vi "Move.vi"(5 "Force":bool, 7 "Valve":string, 10 "max time":i32=26, 11 "Volcano in":refnum<class "Volcano.lvclass">=refnum) -> (1 "Finished?":bool=TRUE, 2 "# elements in queue":i32, 3 "Volcano out":refnum<class "Volcano.lvclass">)   [LabVIEW 2023, in "d16.lvlib" / "Volcano.lvclass"]
uses:
  Volcano.lvclass
  Volcano.lvclass/Volcano.ctl
  <vilib>/Utility/miscctls.llb/LVMapReplaceAction.ctl
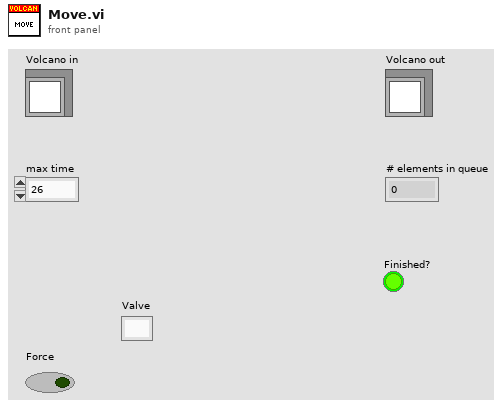
[diagram p1: front panel]
types:
  T1 = typedef "LVMapReplaceAction.ctl" = enum32{"Modify Entry only if found", "Add or Modify Entry", "Delete Entry"}
  T2 = cluster{"Current Valve":string, "Unopened Valves":string[], "Cumulative Pressure Released":u64, "Time":i32}
  T3 = map{string, cluster{"Flow Rate":i32, "Routes":string[], "Route Time":i32[]}}
  T4 = cluster{"Flow Rate":i32, "Routes":string[], "Route Time":i32[]}
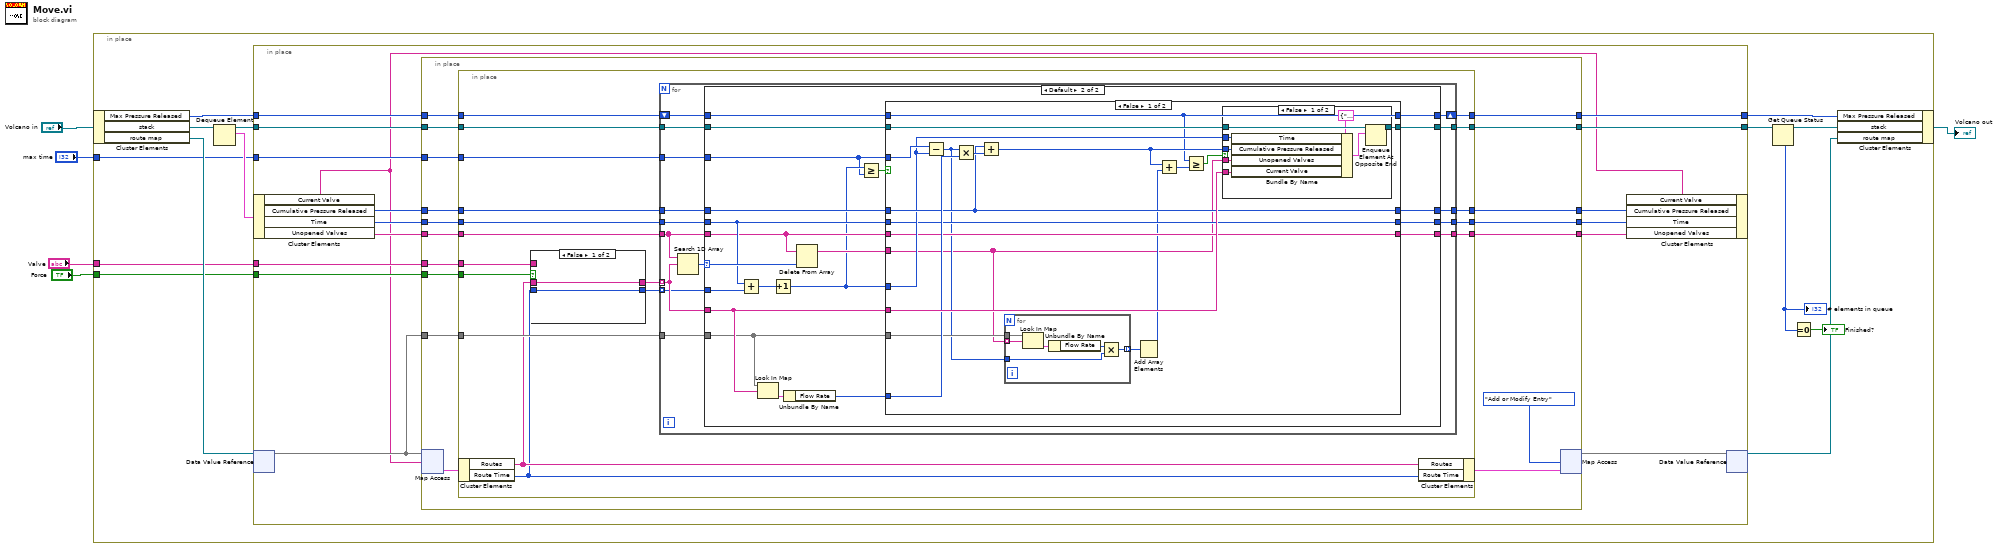
[diagram p0: block diagram]
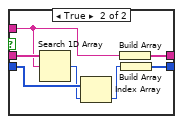
[diagram p2: hidden frame]
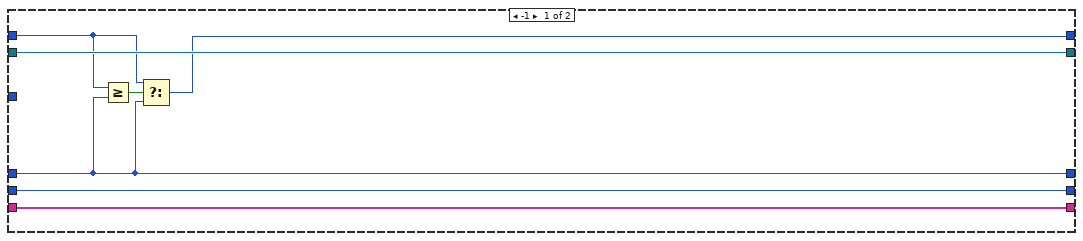
[diagram p3: hidden frame]
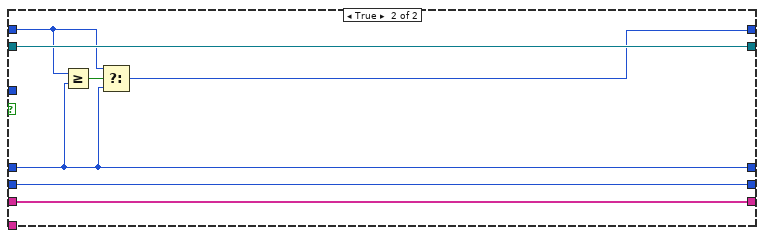
[diagram p5: hidden frame]
diagram:
  n1 = in-place {
    in-place-border: "max time" -> [w15]
    in-place-border: "Force" -> [w7]
    in-place-border: "Valve" -> [w6]
    n2 = in-place-cluster #1("Volcano in") -> ("Max Pressure Released"=w13:u64, "stack"=w19:refnum<queue>, "route map"=w17:refnum<data-value>)
    n3 = Dequeue Element(queue=w19) -> (queue out=w18:refnum<queue>, element=w16:T2)  [unwired: 2 in, 2 out]
    n4 = in-place {
      in-place-border: w18 -> [w35]
      in-place-border: w15 -> [w34]
      in-place-border: [w33] -> w11
      in-place-border: w13 -> [w31]
      in-place-border: [w30] -> w12
      in-place-border: w7 -> [w28]
      in-place-border: w6 -> [w27]
      n5 = in-place-cluster #2(w16) -> ("Current Valve"=w20:string, "Cumulative Pressure Released"=w24:u64, "Time"=w22:i32, "Unopened Valves"=w25:string[])
      n6 = in-place-dvr #3(w17) -> (w29:T3)  [unwired: 1 out]
      n7 = in-place {
        in-place-border: w35 -> [w50]
        in-place-border: w24 -> [w51]
        in-place-border: w34 -> [w44]
        in-place-border: [w49] -> w33
        in-place-border: w22 -> [w45]
        in-place-border: w31 -> [w43]
        in-place-border: [w42] -> w30
        in-place-border: w25 -> [w46]
        in-place-border: w29 -> [w41]
        in-place-border: w28 -> [w40]
        in-place-border: w27 -> [w39]
        in-place-border: [w38] -> w26
        in-place-border: [w37] -> w21
        in-place-border: [w36] -> w23
        n8 = in-place-map #4(w29, w20) -> (w52:T4)  [unwired: 1 in, 1 out]
        n9 = in-place {
          in-place-border: w45 -> [w66]
          in-place-border: w44 -> [w64]
          in-place-border: w51 -> [w65]
          in-place-border: w50 -> [w70]
          in-place-border: [w69] -> w49
          in-place-border: w46 -> [w67]
          in-place-border: w43 -> [w68]
          in-place-border: [w63] -> w42
          in-place-border: w41 -> [w62]
          in-place-border: w40 -> [w61]
          in-place-border: w39 -> [w56]
          in-place-border: [w55] -> w38
          in-place-border: [w54] -> w37
          in-place-border: [w53] -> w36
          n10 = in-place-cluster #5(w52) -> ("Routes"=w60:string[], "Route Time"=w59:i32[])
          n11 = case shown="False" w61 {
            tunnel: w60 -> [w72 w78]
            tunnel: w59 -> [w71 w76]
            tunnel: [w72 w79] -> w58
            tunnel: [w71 w73] -> w57
            tunnel: w56 -> [_ w77]
            frame False {
            }
            frame True {
              n12 = Search 1D Array(1D array=w78, element=w77) -> (index of element=w75:i32)  [unwired: 1 in]
              n13 = Index Array(array=w76, index=w75) -> (element=w74:i32)
              n14 = Build Array(w77) -> (w79:string[])
              n15 = Build Array(w74) -> (w73:i32[])
            }
          }
          n16 = for {
            tunnel: w70 -> [w94]
            tunnel: [w93] -> w69
            tunnel: w67 -> [w92]
            tunnel: w66 -> [w90]
            tunnel: w65 -> [w87]
            tunnel: w64 -> [w88]
            shift-right: [w86] -> w63
            shift-left: w68 -> [w89]
            tunnel: w62 -> [w85]
            tunnel: w58 -> [w84] mode=indexing
            tunnel: w57 -> [w83] mode=indexing
            tunnel: [w82] -> w55
            tunnel: [w81] -> w54
            tunnel: [w80] -> w53
            n17 = Search 1D Array(1D array=w92, element=w84) -> (index of element=w91:i32)  [unwired: 1 in]
            n18 = case shown="Default" w91 {
              selector: w91 -> [_ w120]
              tunnel: w94 -> [w101 w122]
              tunnel: [w101 w121] -> w93
              tunnel: w92 -> [w95 w107]
              tunnel: w90 -> [w96 w109]
              tunnel: w83 -> [_ w118]
              tunnel: w89 -> [w99 w116]
              tunnel: w88 -> [_ w103]
              tunnel: w87 -> [w97 w115]
              tunnel: [w100 w114] -> w86
              tunnel: w85 -> [_ w102]
              tunnel: w84 -> [_ w113]
              tunnel: [w95 w106] -> w82
              tunnel: [w96 w108] -> w81
              tunnel: [w97 w110] -> w80
              frame -1 {
                n19 = Greater Or Equal?(x=w99, y=w97) -> (x >= y?=w98:bool)
                n20 = Select(t=w99, s=w98, f=w97) -> (s? t:f=w100:u64)
              }
              frame Default {
                n21 = Add(x=w109, y=w118) -> (x+y=w105:i32)
                n22 = Look In Map(map=w102, key=w113) -> (value=w112:T4)  [unwired: 1 in, 1 out]
                n23 = Increment(x=w105) -> (x+1=w104:i32)
                n24 = Unbundle By Name(w112) -> ("Flow Rate"=w111:i32)
                n25 = Delete From Array(array=w107, index=w120) -> (array with subset deleted=w119:string[])  [unwired: 1 in, 1 out]
                n26 = Greater Or Equal?(x=w104, y=w103) -> (x >= y?=w117:bool)
                n27 = case shown="False" w117 {
                  tunnel: w122 -> [w141 w163]
                  tunnel: [w140 w163] -> w121
                  tunnel: w119 -> [w123 _]
                  tunnel: w113 -> [w139 _]
                  tunnel: w116 -> [w125 w162]
                  tunnel: w111 -> [w138 _]
                  tunnel: w104 -> [w134 _]
                  tunnel: w103 -> [w137 _]
                  tunnel: w115 -> [w135 w157]
                  tunnel: [w125 w161] -> w114
                  tunnel: [w135 w157] -> w110
                  tunnel: w107 -> [w132 w159]
                  tunnel: w109 -> [w133 w160]
                  tunnel: [w133 w160] -> w108
                  tunnel: [w132 w159] -> w106
                  tunnel: w102 -> [w131 _]
                  frame False {
                    n28 = Subtract(x=w137, y=w134) -> (x-y=w130:i32)
                    n29 = Multiply(x=w130, y=w138) -> (x*y=w136:i32)
                    n30 = Add(x=w135, y=w136) -> (x+y=w127:u64)
                    n31 = for {
                      tunnel: w123 -> [w156] mode=indexing
                      tunnel: w131 -> [w155]
                      tunnel: w130 -> [w152]
                      tunnel: [w151] -> w129 mode=indexing
                      n32 = Look In Map(map=w155, key=w156) -> (value=w154:T4)  [unwired: 1 in, 1 out]
                      n33 = Unbundle By Name(w154) -> ("Flow Rate"=w153:i32)
                      n34 = Multiply(x=w153, y=w152) -> (x*y=w151:i32)
                    }
                    n35 = Add Array Elements(numeric array=w129) -> (sum=w128:i32)
                    n36 = Add(x=w127, y=w128) -> (x+y=w126:u64)
                    n37 = Greater Or Equal?(x=w125, y=w126) -> (x >= y?=w124:bool)
                    n38 = case shown="False" w124 {
                      tunnel: w141 -> [w149 w150]
                      tunnel: [w147 w150] -> w140
                      tunnel: w139 -> [w145 _]
                      tunnel: w127 -> [w144 _]
                      tunnel: w134 -> [w143 _]
                      tunnel: w123 -> [w142 _]
                      frame False {
                        n39 = Bundle By Name(cluster=T2 {"Current Valve"="", "Unopened Valves"=[], "Cumulative Pressure Released"=0, "Time"=0} ("element"), "Time"=w143, "Cumulative Pressure Released"=w144, "Unopened Valves"=w142, "Current Valve"=w145) -> (w148:T2)
                        n40 = Enqueue Element At Opposite End(queue=w149, element=w148) -> (queue out=w147:refnum<queue>)  [unwired: 2 in, 2 out]
                      }
                      frame True {
                      }
                    }
                  }
                  frame True {
                    n41 = Greater Or Equal?(x=w162, y=w157) -> (x >= y?=w158:bool)
                    n42 = Select(t=w162, s=w158, f=w157) -> (s? t:f=w161:u64)
                  }
                }
              }
            }
          }
          n43 = in-place-cluster #5("Routes"=w60, "Route Time"=w59) -> (w48:T4)
        }
        n44 = in-place-map #4(w48, LVMapReplaceAction."Add or Modify Entry" ("action")) -> (w32:T3)  [unwired: 2 out]
      }
      n45 = in-place-cluster #2("Current Valve"=w20, "Cumulative Pressure Released"=w23, "Time"=w21, "Unopened Valves"=w26) -> ()  [unwired: 1 out]
      n46 = in-place-dvr #3(w32) -> (w14:refnum<data-value>)  [unwired: 1 out]
    }
    n47 = Get Queue Status(queue=w11) -> (queue out=w10:refnum<queue>, # elements in queue=w9:i32)  [unwired: 2 in, 6 out]
    "# elements in queue" <- w9
    n48 = Equal To 0?(x=w9) -> (x = 0?=→"Finished?":bool)
    n49 = in-place-cluster #1("Max Pressure Released"=w12, "stack"=w10, "route map"=w14) -> (→"Volcano out":refnum<class "Volcano.lvclass">)
  }
